vi "part2.vi"() -> ()   [LabVIEW 2021]
uses:
  <instrlib>/Tektronix TDS 200 1000 2000 Series/Public/Data/Read (Single Waveform).vi
  <instrlib>/Tektronix TDS 200 1000 2000 Series/Tektronix TDS 200 1000 2000 Series.lvlib
panel:
  in  "Filename 3":path=path "test.lvm" caption="Filename"
  in  "Filename 2":path=path "test.lvm" caption="Filename"
  in  "Filename":path=path "test.lvm"
  in  "error in (no error)":errorcluster
  in  "VISA resource name":refnum<visa-resource-name>
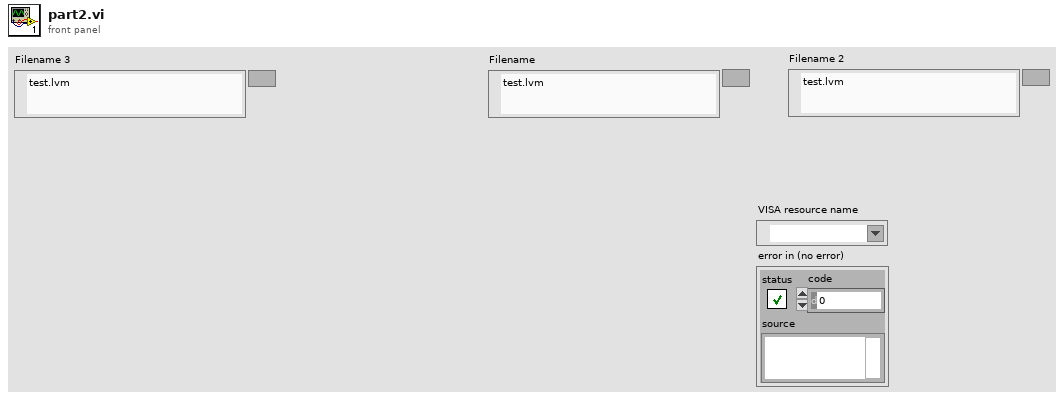
[diagram p1: front panel]
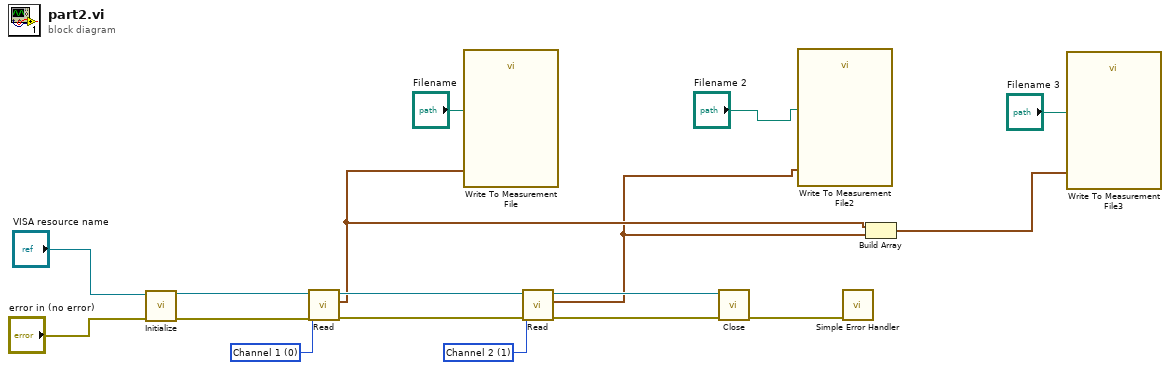
[diagram p0: block diagram]
diagram:
  w9 = u16 1 items=["Channel 1", "Channel 2", "Channel 3", "Channel 4", "Math", "Reference A", "Reference B", "Reference C", "Reference D", "FFT"] ("Source (0: Channel 1)")
  w11 = u16 0 items=["Channel 1", "Channel 2", "Channel 3", "Channel 4", "Math", "Reference A", "Reference B", "Reference C", "Reference D", "FFT"] ("Source (0: Channel 1)")
  n1 = call <instrlib>:"Initialize.vi"("error in (no error)"="error in (no error)", "VISA resource name"="VISA resource name") -> ("error out"=w14:errorcluster, "VISA resource name out"=w15:refnum<visa-resource-name>)  [unwired: 8 in]
  n2 = call-poly <instrlib>:"Read.vi"("error in (no error)"=w14, "Source (0: Channel 1)"=w11, "VISA resource name"=w15) -> ("error out"=w8:errorcluster, "Waveform Data"=w4:waveform(dbl), "VISA resource name out"=w10:refnum<visa-resource-name>)  [unwired: 6 in]
  n3 = call "Write To Measurement File"("Signals"=w4, "Filename"="Filename") -> ()  [unwired: 15 in, 3 out]
  n4 = call-poly <instrlib>:"Read.vi"("error in (no error)"=w8, "Source (0: Channel 1)"=w9, "VISA resource name"=w10) -> ("error out"=w7:errorcluster, "Waveform Data"=w3:waveform(dbl), "VISA resource name out"=w6:refnum<visa-resource-name>)  [unwired: 6 in]
  n5 = call <instrlib>:"Close.vi"("error in (no error)"=w7, "VISA resource name"=w6) -> ("error out"=w13:errorcluster)  [unwired: 9 in]
  n6 = call "Write To Measurement File2"("Signals"=w3, "Filename"="Filename 2") -> ()  [unwired: 15 in, 3 out]
  n7 = call <vilib>:"Simple Error Handler.vi"("error in (no error)"=w13) -> ()  [unwired: 4 in, 5 out]
  n8 = Build Array(w4, w3) -> (w2:waveform(dbl)[])
  n9 = call "Write To Measurement File3"("Signals"=w2, "Filename"="Filename 3") -> ()  [unwired: 15 in, 3 out]
